vi "write-data-wfm-dvr.vi"(7 "wfm size":i32=100, 8 "error in (no error)":errorcluster, 9 "dt":dbl, 10 "data":dbl, 11 "wfm dvr":refnum<data-value>) -> (0 "error out":errorcluster, 3 "wfm dvr":refnum<data-value>)   [LabVIEW 2024]
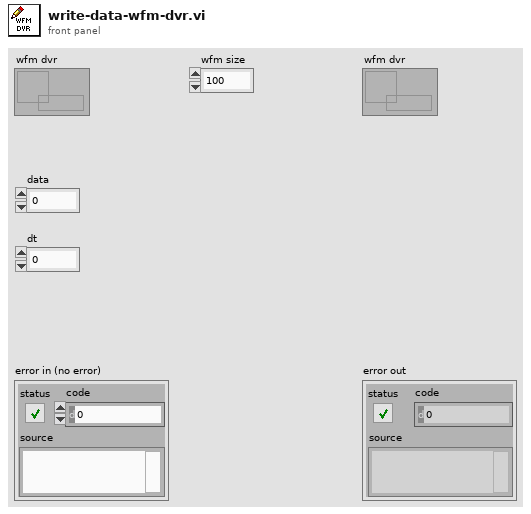
[diagram p1: front panel]
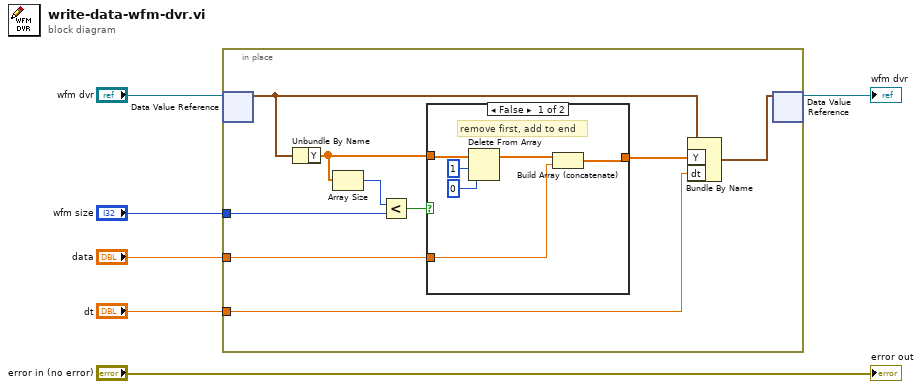
[diagram p0: block diagram]
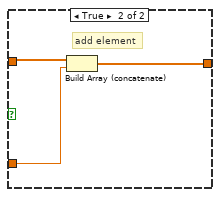
[diagram p2: hidden frame]
diagram:
  n1 = in-place {
    in-place-border: "wfm size" -> [w12]
    in-place-border: "data" -> [w9]
    in-place-border: "dt" -> [w7]
    n2 = in-place-dvr #1("wfm dvr") -> (w15:waveform(dbl))  [unwired: 1 out]
    n3 = Unbundle By Name(w15) -> ("Y"=w10:dbl[])
    n4 = Array Size(array=w10) -> (size(s)=w13:i32)
    n5 = Less?(x=w13, y=w12) -> (x < y?=w11:bool)
    n6 = case shown="False" w11 {
      tunnel: w10 -> [w21 w24]
      tunnel: w9 -> [w17 w23]
      tunnel: [w16 w22] -> w8
      frame False {
        # "remove first, add to end"
        n7 = Delete From Array(array=w21, length=1, index=0) -> (array with subset deleted=w18:dbl[])  [unwired: 1 out]
        n8 = Build Array (concatenate)(w18, w17) -> (w16:dbl[])
      }
      frame True {
        # "add element"
        n9 = Build Array (concatenate)(w24, w23) -> (w22:dbl[])
      }
    }
    n10 = Bundle By Name(cluster=w15, "Y"=w8, "dt"=w7) -> (w14:waveform(dbl))
    n11 = in-place-dvr #1(w14) -> (→"wfm dvr":refnum<data-value>)  [unwired: 1 out]
  }
  "error out" <- "error in (no error)"
